vi "Initialize Sink.vi"(11 "ConsoleSink in":refnum<class "ConsoleSink.lvclass">) -> (0 "error out":errorcluster, 3 "ConsoleSink out":refnum<class "ConsoleSink.lvclass">)   [LabVIEW 2020, in "MVA Framework.lvlib" / "ConsoleView.lvlib" / "ConsoleSink.lvclass"]
uses:
  ConsoleSink.lvclass
  ConsoleSink.lvclass/ConsoleSink.ctl
  <vilib>/ErrorRing/Error Ring.xnode
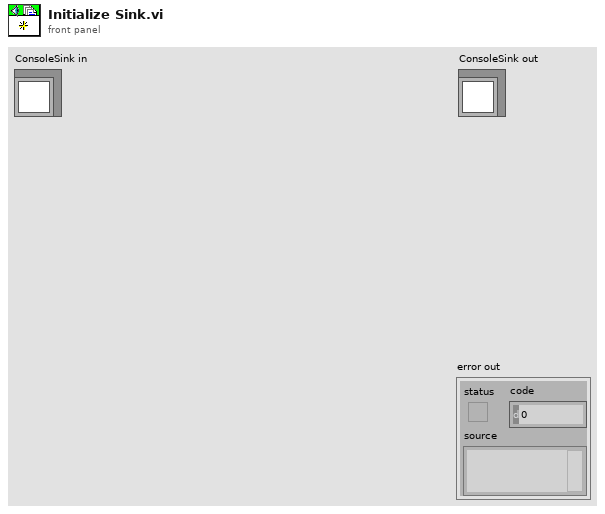
[diagram p1: front panel]
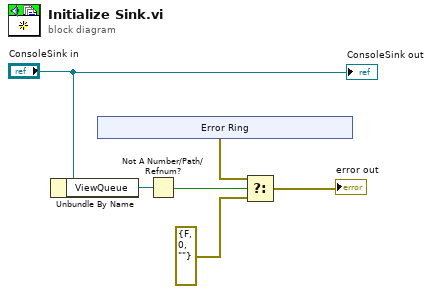
[diagram p0: block diagram]
diagram:
  n1 = Unbundle By Name("ConsoleSink in") -> ("ViewQueue"=w5:refnum<queue>)
  n2 = xnode "Error Ring"() -> ("error out"=w3:errorcluster)
  n3 = Not A Number/Path/Refnum?(number/path/refnum=w5) -> (NaN/Path/Refnum?=w4:bool)
  n4 = Select(t=w3, s=w4, f=errorcluster {"status"=FALSE, "code"=0, "source"=""}) -> (s? t:f=→"error out":errorcluster)
  "ConsoleSink out" <- "ConsoleSink in"
